vi "Destroy.vi"(0 "reference in":refnum<class "SSH.lvclass">, 5 "Error In":errorcluster) -> (14 "reference out":refnum<class "SSH.lvclass">, 19 "Error Out":errorcluster)   [LabVIEW 2023, in "HPS-17000-PowerModule.lvlib" / "SSH.lvclass"]
uses:
  SSH.lvclass
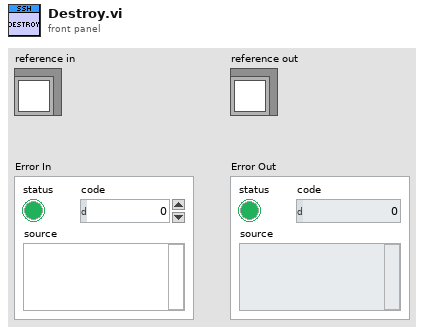
[diagram p1: front panel]
types:
  T1 = typedef "Script.lvclass/ObjectAttributes.ctl" = cluster{"Update Rate (ms)":i32, "Console Listbox":refnum<vi>, "Full Command":string, "Script Name":string, "Log File":string, "IP Address":string, "Script Complete Event":refnum<user-event>}
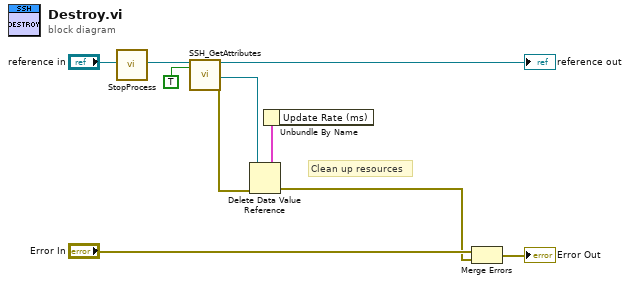
[diagram p0: block diagram]
diagram:
  # "Clean up resources"
  n1 = call "StopProcess.vi"("reference in"="reference in") -> ("reference out"=w1:refnum<class "SSH.lvclass">)  [unwired: 17 in, 1 out]
  n2 = call "SSH_GetAttributes.vi"("reference in"=w1, "OnlyGetDvrReference(False)"=TRUE) -> ("reference out"=→"reference out":refnum<class "SSH.lvclass">, "DataRef"=w7:refnum<data-value>, "Error Out"=w8:errorcluster)  [unwired: 14 in, 1 out]
  n3 = Delete Data Value Reference(data value reference=w7, error in=w8) -> (data value=w3:T1, error out=w5:errorcluster)
  n4 = Unbundle By Name(w3) -> ()  [unwired: 1 out]
  n5 = Merge Errors("Error In", w5) -> (→"Error Out":errorcluster)
